vi "add diagnostics.vi"(8 "error in (no error)":errorcluster, 11 "Item Ref in":T1 format="%.0x") -> (0 "error out":errorcluster, 3 "Parent Ref out":T1 format="%.0x")   [LabVIEW 2021, in "Modbus Master System Explorer.lvlib"]
uses:
  Modbus Master System Explorer.lvlib
  <vilib>/NI VeriStand/Custom Device API/Custom Device Item Ref.ctl
  <vilib>/NI VeriStand/Custom Device API/Custom Device Channel.ctl
  <vilib>/NI VeriStand/Custom Device API/Custom Device Channel Type.ctl
  Shared/Constants.vi
  <vilib>/NI VeriStand/Custom Device API/Custom Device API.lvlib
  Shared/Modbus Master Shared.lvlib
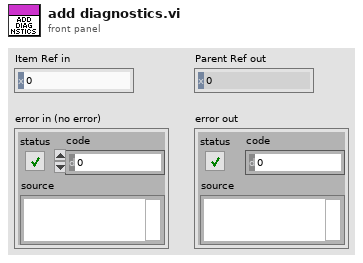
[diagram p1: front panel]
types:
  T1 = typedef "Custom Device API.lvlib/Custom Device Item Ref.ctl" = u64
  T2 = typedef "Custom Device API.lvlib/Custom Device Channel.ctl" = cluster{"Type":T3, "Units":string, "Default Value":dbl, "Faultable":bool, "Scalable":bool}
  T3 = typedef "Custom Device API.lvlib/Custom Device Channel Type.ctl" = enum16{"Input", "Output"}
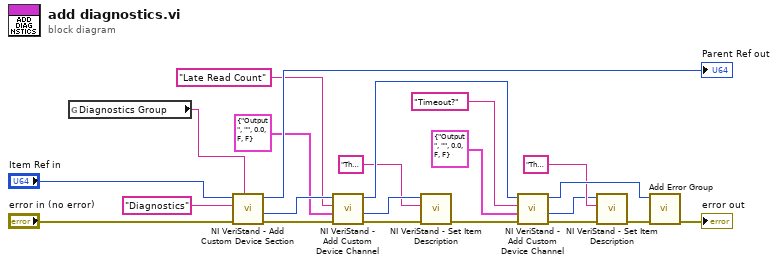
[diagram p0: block diagram]
diagram:
  n1 = global read "Constants.vi" "Diagnostics Group"() -> (w20:string)
  n2 = call <vilib>:"NI VeriStand - Add Custom Device Section.vi"("GUID (Default Section)"=w20, "error in (no error)"="error in (no error)", "Section Name"="Diagnostics", "Parent Ref in"="Item Ref in") -> ("error out"=w19:errorcluster, "Section Ptr"=w22:T1, "Parent Ref out"=→"Parent Ref out":T1)  [unwired: 4 in, 1 out]
  n3 = call <vilib>:"NI VeriStand - Add Custom Device Channel.vi"("error in (no error)"=w19, "Channel"=T2 {"Type"=enum."Output", "Units"="", "Default Value"=0.0, "Faultable"=FALSE, "Scalable"=FALSE}, "Channel Name"="Late Read Count", "Parent Ref in"=w22) -> ("error out"=w4:errorcluster, "Channel Ref"=w8:T1, "Parent Ref out"=w11:T1)  [unwired: 4 in, 1 out]
  n4 = call <vilib>:"NI VeriStand - Set Item Description.vi"("error in (no error)"=w4, "Description"="The Late Read Count channel is incremented any time the read loop in the engine returns late. ", "Item Ref in"=w8) -> ("error out"=w3:errorcluster)  [unwired: 6 in, 2 out]
  n5 = call <vilib>:"NI VeriStand - Add Custom Device Channel.vi"("error in (no error)"=w3, "Channel"=T2 {"Type"=enum."Output", "Units"="", "Default Value"=0.0, "Faultable"=FALSE, "Scalable"=FALSE}, "Channel Name"="Timeout?", "Parent Ref in"=w11) -> ("error out"=w2:errorcluster, "Channel Ref"=w5:T1, "Parent Ref out"=w15:T1)  [unwired: 4 in, 1 out]
  n6 = call <vilib>:"NI VeriStand - Set Item Description.vi"("error in (no error)"=w2, "Description"="The Timeout? channel is asserted any time a read or write command times out. It is deasserted when a read or write is successfully executed without timing out.", "Item Ref in"=w5) -> ("error out"=w1:errorcluster)  [unwired: 6 in, 2 out]
  n7 = call "Add Error Group.vi"("error in (no error)"=w1, "Parent Ref in"=w15) -> ("error out"=→"error out":errorcluster)  [unwired: 8 in, 1 out]
